vi "integer-string converter.vi"(3 "integer string in":string[](array[string]), 5 "integer in":i32[](array[numeric])) -> (0 "integer out":i32[](array[numeric]), 2 "integer string out":string[](array[string]))   [LabVIEW 2015]
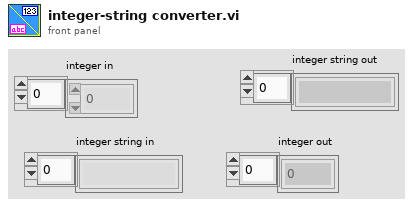
[diagram p1: front panel]
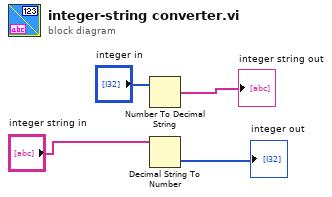
[diagram p0: block diagram]
diagram:
  n1 = Number To Decimal String(number="integer in") -> (decimal integer string=→"integer string out":string[])  [unwired: 1 in]
  n2 = Decimal String To Number(string="integer string in") -> (number=→"integer out":i32[])  [unwired: 2 in, 1 out]
